vi "write_converter_file.vi"(9 "CONVERTER":cluster{u16, u16, i16}, 10 "minutes":dbl, 11 "converter file":path) -> ()   [LabVIEW 2019]
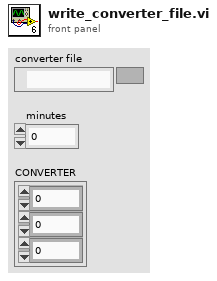
[diagram p1: front panel]
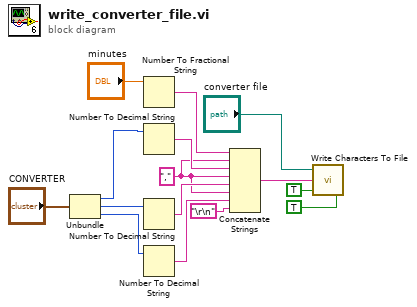
[diagram p0: block diagram]
diagram:
  w2 = "," ("string")
  n1 = Unbundle("CONVERTER") -> (w1:u16, w9:u16, w10:i16)
  n2 = Number To Fractional String(number="minutes") -> (F-format string=w11:string)  [unwired: 3 in]
  n3 = Number To Decimal String(number=w1) -> (decimal integer string=w12:string)  [unwired: 1 in]
  n4 = Number To Decimal String(number=w9) -> (decimal integer string=w13:string)  [unwired: 1 in]
  n5 = Number To Decimal String(number=w10) -> (decimal integer string=w3:string)  [unwired: 1 in]
  n6 = Concatenate Strings(w11, w2, w12, w2, w13, w2, w3, "\r\n") -> (w14:string)
  n7 = call <vilib>:"Write Characters To File.vi"("convert eol? (no:F)"=TRUE, "append to file? (new file:F)"=TRUE, "character string"=w14, "file path (dialog if empty)"="converter file") -> ()  [unwired: 1 in, 1 out]
